vi "PurePursuit.vi"(0 "PathData":T2={"Path"=[{"x"=0.0, "y"=0.0}, {"x"=0.0, "y"=46.0}, {"x"=77.25, "y"=97.5}], "Spacing"=0.0, "DistancesToEnd"=[309.52253206522465, 306.5225388483889, 303.52254576348514, 300.5225494135135, 297.5225482930251, 294.5225431892043, 291.52253649479525, 288.5225309404311, 285.52252839669825, 282.52252922985826, 279.52253236801363, 276.5225359199274, 273.5225380077533, 270.5225374640896, 267.5225341651582, 264.5225289486152, 261.52252321975885, 258.52251843460203, 255.52251565052453, 252.52251527415513, 249.52251704698162, 246.52252022727612, 243.52252387624657, 240.5225271449837, 237.52252948071848, 234.5225307115883, 231.5225310121264, 228.5225307841412, 225.52253050297352, 222.52253057724883, 219.522531255923, 216.52253259658312, 213.5225344902357, 210.52253672481638, 207.52253906428678, 204.52254132188853, 201.52254341264756, 198.5225453787386, 195.52254738922483, 192.52254972128023, 189.5225527326013, 186.5225568345679, 183.5225624736694, 180.52257012582595, 177.52258030545136, 174.52259358906986, 171.52261065227918, 168.52263231879937, 165.52265962102405, 162.52269387257934, 159.52273675466557, 156.52279041923995, 153.52285761342083, 150.52294183093122, 147.52304749810799, 144.52318020416902, 141.5233469881785, 138.52355669860665, 135.52382044572104, 132.52415217017628, 129.52456938475245, 126.52509392552396, 123.52575388229783, 120.52658224756205, 117.52762599636499, 114.52893466674816, 111.5305811433295, 108.53265099247815, 105.5352499693053, 102.53851522329074, 99.54261858949184, 96.54777258499563, 93.55424339621041, 90.56236601643654, 87.57255952674781, 84.58534501572932, 81.60137180227034, 78.62143961905741, 75.64655567097594, 72.6779255489502, 69.71706974165639, 66.76578984976493, 63.82625595622302, 60.90103565379168, 57.99306437227732, 55.10557379235981, 52.24189700353533, 49.40502603383819, 46.59675379579783, 43.81612021857386, 41.056705992040605, 38.30212773163372, 35.53590323835957, 32.752089130751756, 29.950811925036337, 27.135602619179224, 24.311917874683846, 21.486403150766286, 18.666614193530503, 15.861028930660632, 13.07925664424869, 10.33239795871144, 7.633538890247935, 4.998382632368401, 2.4460384085185156, 0.0]}, 1 "SensorData":T3, 3 "Trackwidth":dbl=40.0 format="%#_13g", 5 "LookAhead":dbl=30.0, 9 "MaxVel":dbl=85.0, 11 "error in (no error)":errorcluster, 12 "Max Accel":dbl=65.0 format="%#_13g", 14 "Gains":T4={"FFV"=0.0088, "FFA"=0.0017, "Vel PID"={"P"=0.01, "I"=0.007, "D"=0.0}} {"Vel PID"."D" format="%.3f"; "Vel PID"."I" format="%.3f"; "Vel PID"."P" format="%.3f"}) -> (2 "Graph":cluster{cluster{"x":dbl, "y":dbl}[]}[](graph)=[{[{"x"=0.0, "y"=0.0}, {"x"=6.123233995736766e-17, "y"=1.0}, {"x"=1.2246467991473532e-16, "y"=2.0}, {"x"=1.8369701987210297e-16, "y"=3.0}, {"x"=2.4492935982947064e-16, "y"=4.0}, {"x"=3.061616997868383e-16, "y"=5.0}, {"x"=3.6739403974420594e-16, "y"=6.0}, {"x"=4.286263797015736e-16, "y"=7.0}, {"x"=4.898587196589413e-16, "y"=8.0}, {"x"=5.51091059616309e-16, "y"=9.0}, {"x"=6.123233995736766e-16, "y"=10.0}, {"x"=6.735557395310443e-16, "y"=11.0}, {"x"=7.347880794884119e-16, "y"=12.0}, {"x"=7.960204194457795e-16, "y"=13.0}, {"x"=8.572527594031472e-16, "y"=14.0}, {"x"=9.18485099360515e-16, "y"=15.0}, {"x"=9.797174393178826e-16, "y"=16.0}, {"x"=1.0409497792752501e-15, "y"=17.0}, {"x"=1.102182119232618e-15, "y"=18.0}, {"x"=1.1634144591899855e-15, "y"=19.0}, {"x"=1.2246467991473533e-15, "y"=20.0}, {"x"=1.2858791391047208e-15, "y"=21.0}, {"x"=1.3471114790620886e-15, "y"=22.0}, {"x"=1.4083438190194562e-15, "y"=23.0}, {"x"=1.4695761589768238e-15, "y"=24.0}, {"x"=1.5308084989341915e-15, "y"=25.0}, {"x"=1.592040838891559e-15, "y"=26.0}, {"x"=1.6532731788489269e-15, "y"=27.0}, {"x"=1.7145055188062944e-15, "y"=28.0}, {"x"=1.7757378587636622e-15, "y"=29.0}, {"x"=1.83697019872103e-15, "y"=30.0}, {"x"=1.8982025386783976e-15, "y"=31.0}, {"x"=1.959434878635765e-15, "y"=32.0}, {"x"=2.0206672185931327e-15, "y"=33.0}, {"x"=2.0818995585505003e-15, "y"=34.0}, {"x"=2.1431318985078682e-15, "y"=35.0}, {"x"=2.204364238465236e-15, "y"=36.0}, {"x"=2.2655965784226034e-15, "y"=37.0}, {"x"=2.326828918379971e-15, "y"=38.0}, {"x"=2.388061258337339e-15, "y"=39.0}, {"x"=2.4492935982947065e-15, "y"=40.0}, {"x"=2.510525938252074e-15, "y"=41.0}, {"x"=2.5717582782094417e-15, "y"=42.0}, {"x"=2.6329906181668092e-15, "y"=43.0}, {"x"=2.6942229581241772e-15, "y"=44.0}, {"x"=2.7554552980815448e-15, "y"=45.0}, {"x"=0.0, "y"=46.0}, {"x"=0.8320502943378437, "y"=46.55470019622523}, {"x"=1.6641005886756874, "y"=47.10940039245046}, {"x"=2.4961508830135313, "y"=47.66410058867569}, {"x"=3.328201177351375, "y"=48.218800784900914}, {"x"=4.160251471689219, "y"=48.77350098112615}, {"x"=4.9923017660270625, "y"=49.328201177351374}, {"x"=5.824352060364906, "y"=49.8829013735766}, {"x"=6.65640235470275, "y"=50.437601569801835}, {"x"=7.488452649040593, "y"=50.99230176602706}, {"x"=8.320502943378438, "y"=51.54700196225229}, {"x"=9.152553237716281, "y"=52.10170215847752}, {"x"=9.984603532054125, "y"=52.65640235470275}, {"x"=10.816653826391969, "y"=53.211102550927976}, {"x"=11.648704120729812, "y"=53.76580274715321}, {"x"=12.480754415067656, "y"=54.320502943378436}, {"x"=13.3128047094055, "y"=54.87520313960366}, {"x"=14.144855003743343, "y"=55.4299033358289}, {"x"=14.976905298081187, "y"=55.98460353205412}, {"x"=15.80895559241903, "y"=56.53930372827935}, {"x"=16.641005886756876, "y"=57.09400392450458}, {"x"=17.47305618109472, "y"=57.64870412072981}, {"x"=18.305106475432563, "y"=58.20340431695504}, {"x"=19.137156769770407, "y"=58.75810451318027}, {"x"=19.96920706410825, "y"=59.3128047094055}, {"x"=20.801257358446094, "y"=59.867504905630724}, {"x"=21.633307652783937, "y"=60.42220510185595}, {"x"=22.46535794712178, "y"=60.976905298081185}, {"x"=23.297408241459625, "y"=61.53160549430641}, {"x"=24.12945853579747, "y"=62.086305690531645}, {"x"=24.961508830135312, "y"=62.64100588675687}, {"x"=25.793559124473155, "y"=63.1957060829821}, {"x"=26.625609418811, "y"=63.750406279207326}, {"x"=27.457659713148843, "y"=64.30510647543255}, {"x"=28.289710007486686, "y"=64.8598066716578}, {"x"=29.12176030182453, "y"=65.41450686788302}, {"x"=29.953810596162374, "y"=65.96920706410825}, {"x"=30.785860890500217, "y"=66.52390726033347}, {"x"=31.61791118483806, "y"=67.0786074565587}, {"x"=32.449961479175904, "y"=67.63330765278394}, {"x"=33.28201177351375, "y"=68.18800784900915}, {"x"=34.11406206785159, "y"=68.7427080452344}, {"x"=34.94611236218944, "y"=69.29740824145962}, {"x"=35.77816265652728, "y"=69.85210843768485}, {"x"=36.610212950865126, "y"=70.40680863391007}, {"x"=37.442263245202966, "y"=70.9615088301353}, {"x"=38.27431353954081, "y"=71.51620902636054}, {"x"=39.10636383387865, "y"=72.07090922258577}, {"x"=39.9384141282165, "y"=72.625609418811}, {"x"=40.77046442255434, "y"=73.18030961503622}, {"x"=41.60251471689219, "y"=73.73500981126145}, {"x"=42.43456501123003, "y"=74.28971000748668}, {"x"=43.266615305567875, "y"=74.8444102037119}, {"x"=44.098665599905715, "y"=75.39911039993714}, {"x"=44.93071589424356, "y"=75.95381059616237}, {"x"=45.7627661885814, "y"=76.5085107923876}, {"x"=46.59481648291925, "y"=77.06321098861282}, {"x"=47.42686677725709, "y"=77.61791118483805}, {"x"=48.25891707159494, "y"=78.17261138106329}, {"x"=49.09096736593278, "y"=78.7273115772885}, {"x"=49.923017660270624, "y"=79.28201177351374}, {"x"=50.755067954608464, "y"=79.83671196973897}, {"x"=51.58711824894631, "y"=80.3914121659642}, {"x"=52.41916854328415, "y"=80.94611236218944}, {"x"=53.251218837622, "y"=81.50081255841465}, {"x"=54.083269131959845, "y"=82.05551275463989}, {"x"=54.915319426297685, "y"=82.61021295086512}, {"x"=55.74736972063553, "y"=83.16491314709035}, {"x"=56.57942001497337, "y"=83.71961334331557}, {"x"=57.41147030931122, "y"=84.2743135395408}, {"x"=58.24352060364906, "y"=84.82901373576604}, {"x"=59.07557089798691, "y"=85.38371393199125}, {"x"=59.90762119232475, "y"=85.9384141282165}, {"x"=60.739671486662594, "y"=86.49311432444172}, {"x"=61.571721781000434, "y"=87.04781452066695}, {"x"=62.40377207533828, "y"=87.60251471689219}, {"x"=63.23582236967612, "y"=88.1572149131174}, {"x"=64.06787266401396, "y"=88.71191510934264}, {"x"=64.89992295835181, "y"=89.26661530556787}, {"x"=65.73197325268966, "y"=89.8213155017931}, {"x"=66.5640235470275, "y"=90.37601569801832}, {"x"=67.39607384136534, "y"=90.93071589424355}, {"x"=68.22812413570318, "y"=91.48541609046879}, {"x"=69.06017443004103, "y"=92.040116286694}, {"x"=69.89222472437888, "y"=92.59481648291924}, {"x"=70.72427501871671, "y"=93.14951667914447}, {"x"=71.55632531305456, "y"=93.7042168753697}, {"x"=72.3883756073924, "y"=94.25891707159494}, {"x"=73.22042590173025, "y"=94.81361726782015}, {"x"=74.05247619606808, "y"=95.36831746404539}, {"x"=74.88452649040593, "y"=95.92301766027062}, {"x"=75.71657678474378, "y"=96.47771785649584}, {"x"=76.54862707908163, "y"=97.03241805272107}, {"x"=77.25, "y"=97.5}]}, {[{"x"=77.17737509961091, "y"=96.61921805961741}, {"x"=87.19208931316219, "y"=103.23023153872136}]}, {[{"x"=77.25, "y"=97.5}]}, {[{"x"=106.17737509961091, "y"=96.61921805961741}, {"x"=104.75801407217037, "y"=105.58071089649088}, {"x"=100.63886793648439, "y"=113.66499037609913}, {"x"=94.22314741609263, "y"=120.08071089649088}, {"x"=86.13886793648439, "y"=124.19985703217687}, {"x"=77.17737509961091, "y"=125.61921805961741}, {"x"=68.21588226273744, "y"=124.19985703217687}, {"x"=60.131602783129196, "y"=120.08071089649088}, {"x"=53.71588226273744, "y"=113.66499037609913}, {"x"=49.59673612705146, "y"=105.58071089649088}, {"x"=48.17737509961091, "y"=96.61921805961741}, {"x"=49.59673612705146, "y"=87.65772522274393}, {"x"=53.71588226273744, "y"=79.5734457431357}, {"x"=60.13160278312919, "y"=73.15772522274393}, {"x"=68.21588226273744, "y"=69.03857908705795}, {"x"=77.17737509961091, "y"=67.61921805961741}, {"x"=86.13886793648439, "y"=69.03857908705795}, {"x"=94.22314741609263, "y"=73.15772522274393}, {"x"=100.63886793648439, "y"=79.57344574313568}, {"x"=104.75801407217037, "y"=87.65772522274393}, {"x"=106.17737509961091, "y"=96.61921805961741}]}, {[{"x"=-861.1099608069076, "y"=601.5180796852112}, {"x"=-831.4997189012965, "y"=414.5663700037659}, {"x"=-745.5674499688715, "y"=245.9147962350945}, {"x"=-611.7248032180614, "y"=112.07214948428447}, {"x"=-443.07322944939017, "y"=26.13988055185939}, {"x"=-256.12151976794485, "y"=-3.470361353751514}, {"x"=-69.1698100864995, "y"=26.13988055185939}, {"x"=99.48176368217185, "y"=112.07214948428447}, {"x"=233.3244104329819, "y"=245.9147962350944}, {"x"=319.256679365407, "y"=414.56637000376577}, {"x"=348.86692127101793, "y"=601.5180796852111}, {"x"=319.256679365407, "y"=788.4697893666564}, {"x"=233.324410432982, "y"=957.1213631353278}, {"x"=99.48176368217202, "y"=1090.9640098861378}, {"x"=-69.16981008649935, "y"=1176.8962788185631}, {"x"=-256.1215197679447, "y"=1206.506520724174}, {"x"=-443.07322944939006, "y"=1176.8962788185631}, {"x"=-611.7248032180614, "y"=1090.964009886138}, {"x"=-745.5674499688714, "y"=957.121363135328}, {"x"=-831.4997189012965, "y"=788.4697893666566}, {"x"=-861.1099608069076, "y"=601.5180796852113}]}], 4 "LeftValue":dbl, 6 "RightValue":dbl, 10 "Done":bool, 15 "error out":errorcluster)   [LabVIEW 2017]
doc: "Takes in encoder and gyro data, and a path. In real time, calculates the left and right power to send to the motors to travel the path at a specified max speed, acceleration, and lookahead distance"
panel:
  out "Waveform Chart":T1(graph)
  in  "Average Vels":bool
  # "SET DEFAULTS"
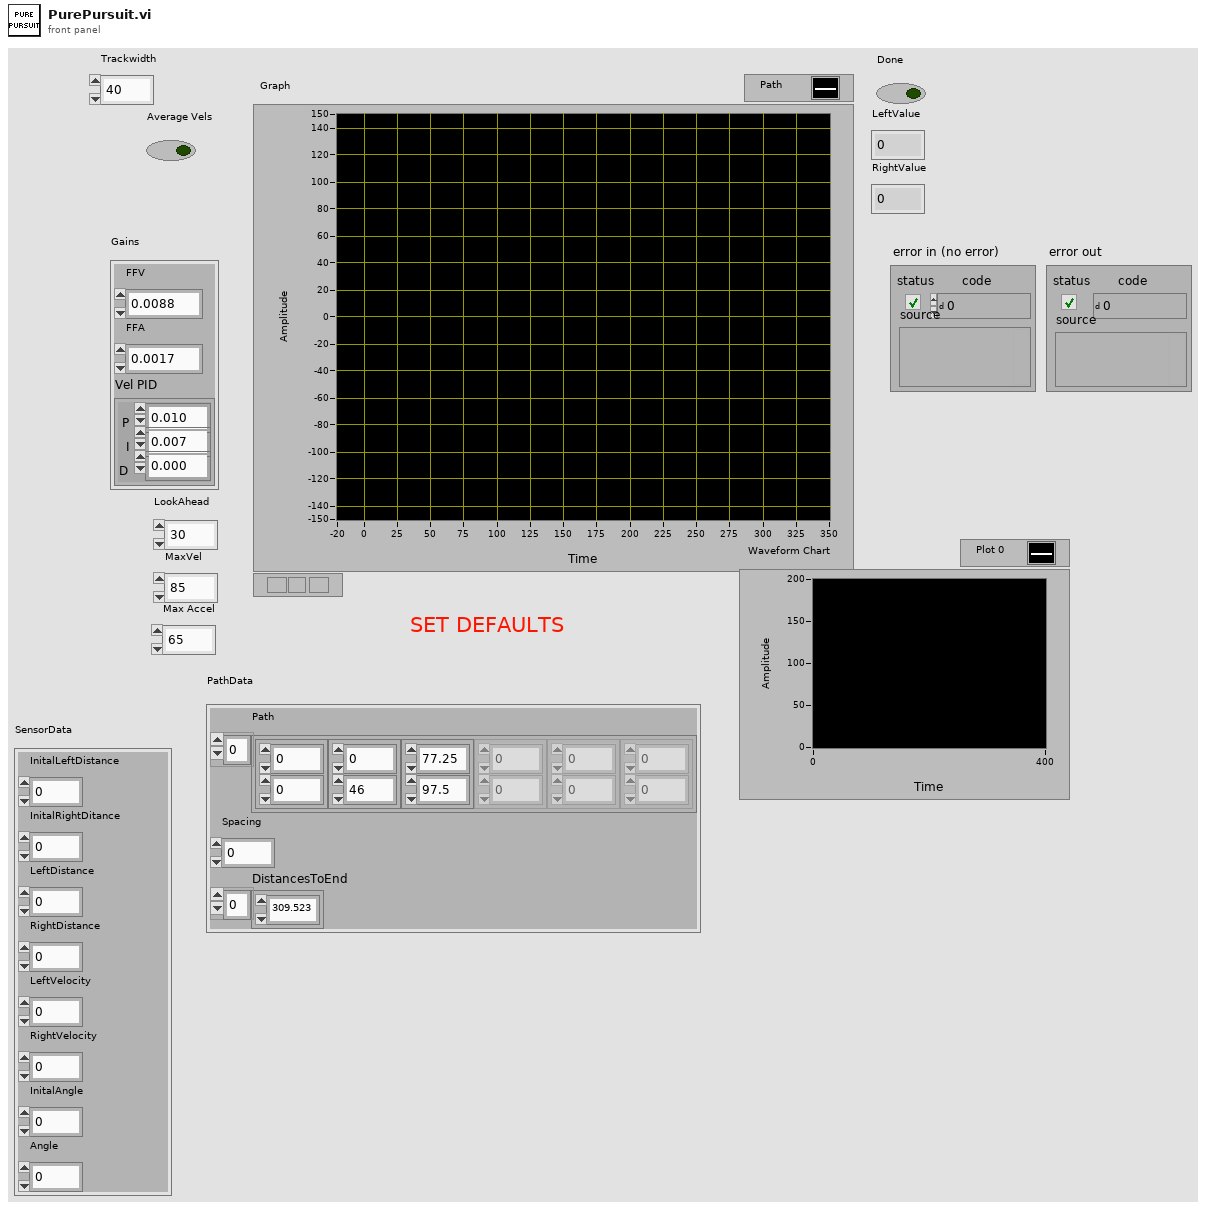
[diagram p1: front panel]
types:
  T1 = cluster{"l":dbl, "dx/dt":dbl, "r":dbl, "dx/dt":dbl}
  T2 = cluster{"Path":cluster{"x":dbl, "y":dbl}[], "Spacing":dbl, "DistancesToEnd":dbl[]}
  T3 = cluster{"InitalLeftDistance":dbl, "InitalRightDitance":dbl, "LeftDistance":dbl, "RightDistance":dbl, "LeftVelocity":dbl, "RightVelocity":dbl, "InitalAngle":dbl, "Angle":dbl}
  T4 = cluster{"FFV":dbl, "FFA":dbl, "Vel PID":cluster{"P":dbl, "I":dbl, "D":dbl}}
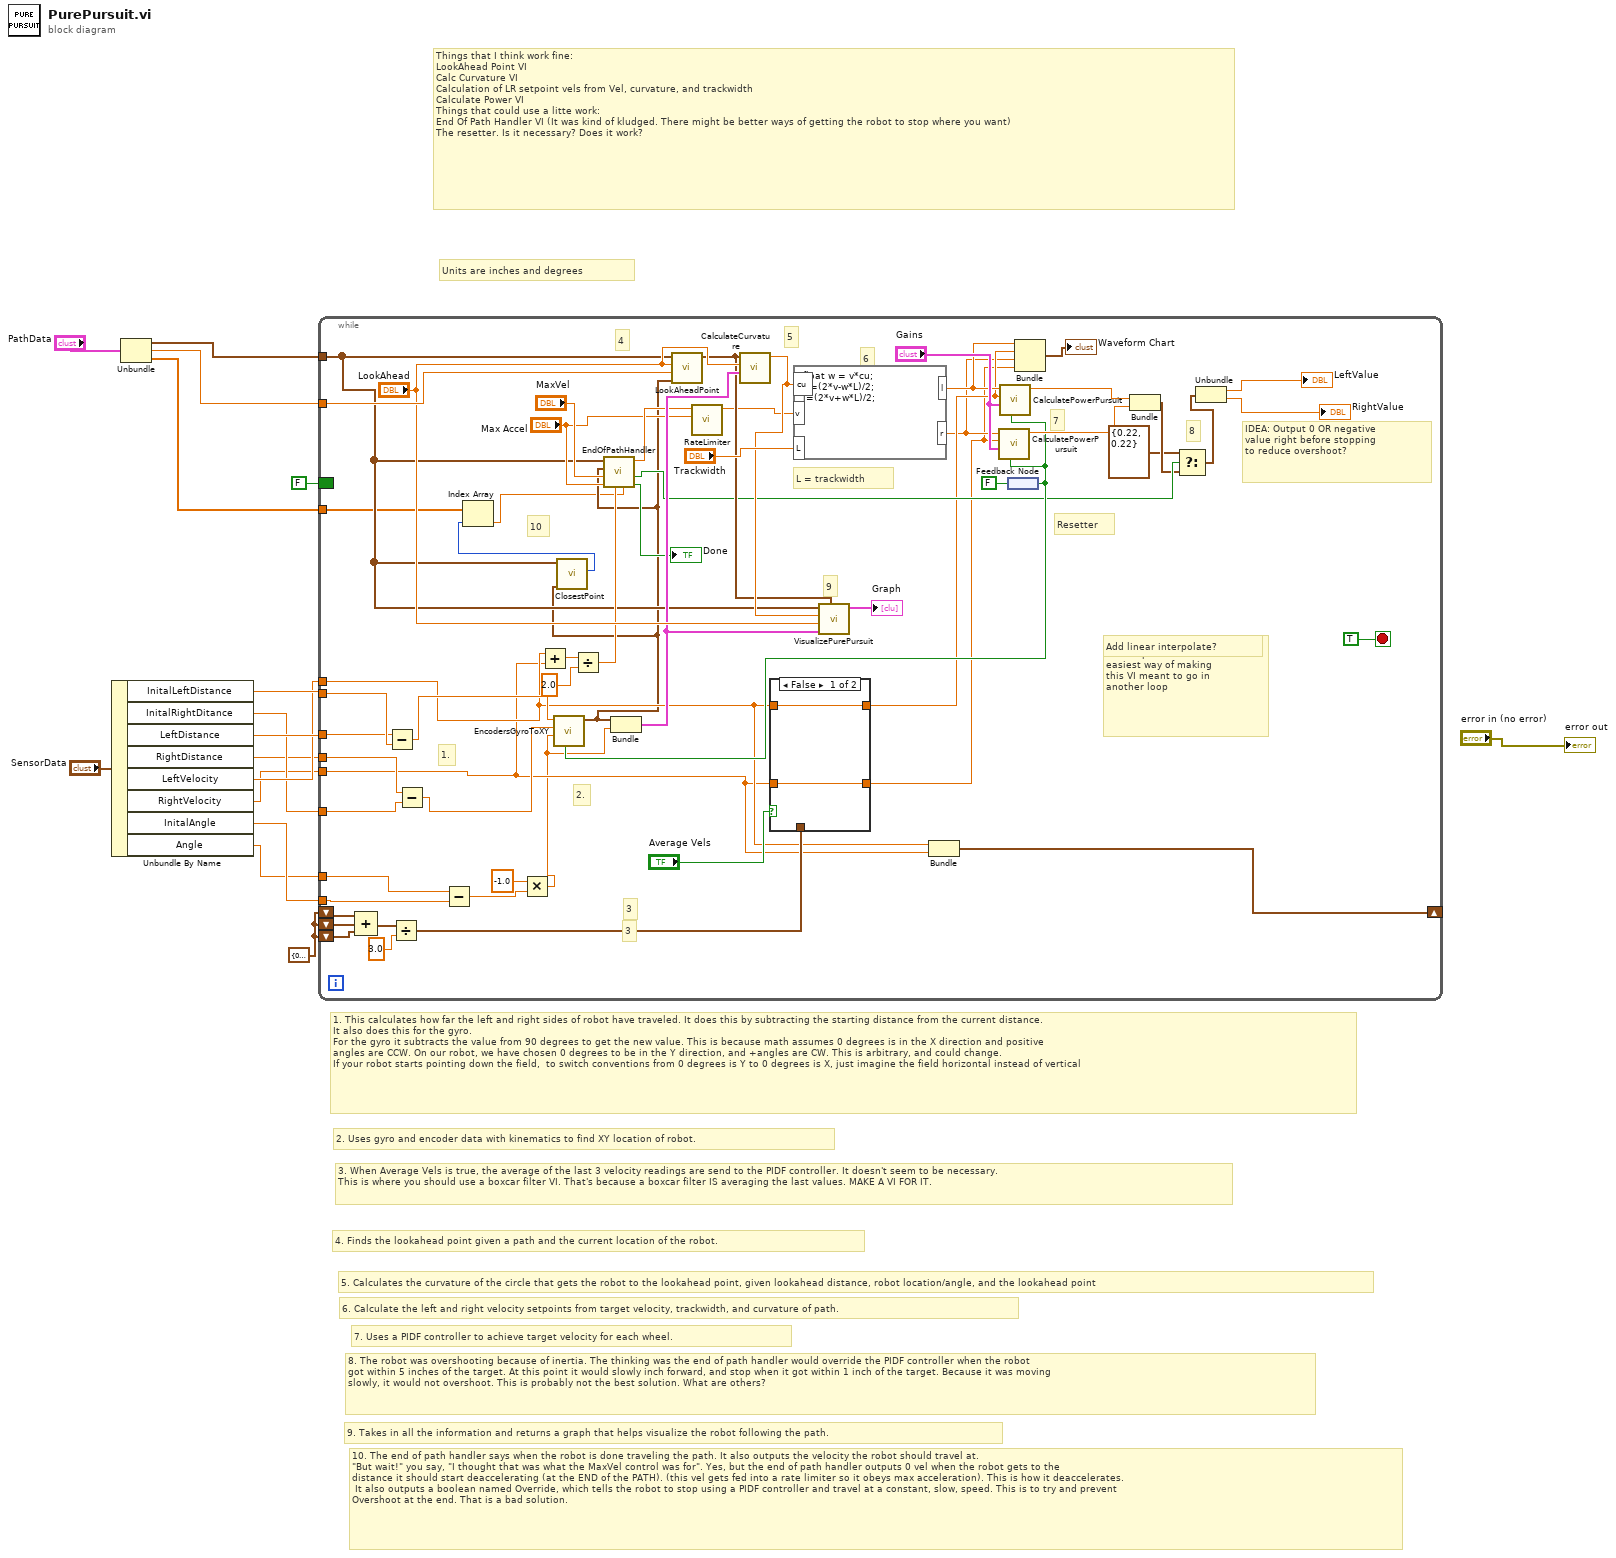
[diagram p0: block diagram]
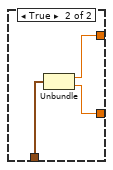
[diagram p2: hidden frame]
diagram:
  w16 = cluster{"dx/dt":dbl, "dx/dt":dbl} {"dx/dt"=0.0, "dx/dt"=0.0}
  # "10. The end of path handler says when the robot is done traveling the path. It also outputs the velocity the robot should travel at.\n\"But wait!\" you say, \"I thought that was what the MaxVel control was for\". Yes, but the end of path handler outputs 0 vel when the robot gets to the\ndistance it should start deaccelerating (at the END of the PATH). (this vel gets fed into a rate limiter so it obeys max acceleration). This is how it deaccelerates. \n It also outputs a boolean named Override, which tells the robot to stop using a PIDF controller and travel at a constant, slow, speed. This is to try and prevent\nOvershoot at the end. That is a bad solution."
  # "9. Takes in all the information and returns a graph that helps visualize the robot following the path."
  # "8. The robot was overshooting because of inertia. The thinking was the end of path handler would override the PIDF controller when the robot\ngot within 5 inches of the target. At this point it would slowly inch forward, and stop when it got within 1 inch of the target. Because it was moving\nslowly, it would not overshoot. This is probably not the best solution. What are others?"
  # "7. Uses a PIDF controller to achieve target velocity for each wheel."
  # "6. Calculate the left and right velocity setpoints from target velocity, trackwidth, and curvature of path."
  # "Things that I think work fine:\nLookAhead Point VI\nCalc Curvature VI\nCalculation of LR setpoint vels from Vel, curvature, and trackwidth\nCalculate Power VI\nThings that could use a litte work:\nEnd Of Path Handler VI (It was kind of kludged. There might be better ways of getting the robot to stop where you want)\nThe resetter. Is it necessary? Does it work?"
  # "Units are inches and degrees"
  # "5. Calculates the curvature of the circle that gets the robot to the lookahead point, given lookahead distance, robot location/angle, and the lookahead point"
  # "4. Finds the lookahead point given a path and the current location of the robot."
  # "3. When Average Vels is true, the average of the last 3 velocity readings are send to the PIDF controller. It doesn't seem to be necessary.\nThis is where you should use a boxcar filter VI. That's because a boxcar filter IS averaging the last values. MAKE A VI FOR IT."
  # "2. Uses gyro and encoder data with kinematics to find XY location of robot."
  # "1. This calculates how far the left and right sides of robot have traveled. It does this by subtracting the starting distance from the current distance.\nIt also does this for the gyro.\nFor the gyro it subtracts the value from 90 degrees to get the new value. This is because math assumes 0 degrees is in the X direction and positive\nangles are CCW. On our robot, we have chosen 0 degrees to be in the Y direction, and +angles are CW. This is arbitrary, and could change.\nIf your robot starts pointing down the field,  to switch conventions from 0 degrees is Y to 0 degrees is X, just imagine the field horizontal instead of vertical"
  n1 = Unbundle By Name("SensorData") -> ("InitalLeftDistance"=w12:dbl, "InitalRightDitance"=w9:dbl, "LeftDistance"=w11:dbl, "RightDistance"=w8:dbl, "LeftVelocity"=w10:dbl, "RightVelocity"=w7:dbl, "InitalAngle"=w6:dbl, "Angle"=w5:dbl)
  n2 = Unbundle("PathData") -> ("Path"=w3:cluster{"x":dbl, "y":dbl}[], "Spacing"=w2:dbl, "DistancesToEnd"=w1:dbl[])
  n3 = while {
    tunnel: w3 -> [w22]
    tunnel: w2 -> [w73]
    shift-right: [w65] -> _
    shift-left: w16 -> [w64]
    shift-left: w16 -> [w63]
    shift-left: w16 -> [w62]
    border: FALSE ("ENABLE") -> [_]
    tunnel: w6 -> [w51]
    tunnel: w9 -> [w50]
    tunnel: w12 -> [w49]
    tunnel: w11 -> [w35]
    tunnel: w10 -> [w34]
    tunnel: w8 -> [w33]
    tunnel: w7 -> [w32]
    tunnel: w5 -> [w31]
    tunnel: w1 -> [w19]
    stop <- TRUE stop-if-true
    # "IDEA: Output 0 OR negative\nvalue right before stopping\nto reduce overshoot?"
    # "10"
    # "9"
    # "8"
    # "7"
    # "6"
    # "5"
    # "4"
    # "3"
    # "3"
    # "2."
    # "1."
    # "I already had everything\nin a loop so this was the\neasiest way of making\nthis VI meant to go in\nanother loop"
    # "Resetter"
    # "Add linear interpolate?"
    # "L = trackwidth"
    n4 = Compound Arithmetic op=ADD(w64, w63, w62) -> (w61:cluster{"dx/dt":dbl, "dx/dt":dbl})
    n5 = Subtract(x=w35, y=w49) -> (x-y=w70:dbl)
    n6 = Divide(x=w61, y=3.0 ("x")) -> (x/y=w58:cluster{"dx/dt":dbl, "dx/dt":dbl})
    n7 = Subtract(x=w33, y=w50) -> (x-y=w74:dbl)
    n8 = Subtract(x=w31, y=w51) -> (x-y=w25:dbl)
    n9 = Multiply(x=-1.0, y=w25) -> (x*y=w27:dbl)
    n10 = Add(x=w34, y=w32) -> (x+y=w41:dbl)
    n11 = Divide(x=w41, y=2.0) -> (x/y=w39:dbl)
    n12 = case shown="False" "Average Vels" {
      tunnel: w32 -> [w76 _]
      tunnel: [w76 w78] -> w23
      tunnel: w34 -> [w75 _]
      tunnel: [w75 w79] -> w28
      tunnel: w58 -> [_ w77]
      frame False {
      }
      frame True {
        n13 = Unbundle(w77) -> ("dx/dt"=w79:dbl, "dx/dt"=w78:dbl)
      }
    }
    n14 = Bundle("LeftVelocity"=w34, "RightVelocity"=w32) -> (w65:cluster{"LeftVelocity":dbl, "RightVelocity":dbl})  [unwired: 1 in]
    n15 = feedback-in #1(FALSE ("ENABLE")) -> ()
    n16 = feedback #1() -> (w54:bool)
    n17 = call "EncodersGyroToXY.vi"("Reset"=w54, "Angle (degrees)"=w27, "Right Distance"=w74, "Left Distance"=w70) -> ("Location"=w21:cluster{dbl, dbl})  [unwired: 6 in, 1 out]
    n18 = call "ClosestPoint.vi"("Robot"=w21, "Path"=w22) -> ("ClosestIndex"=w18:i32)  [unwired: 8 in, 1 out]
    n19 = Index Array(array=w19, index=w18) -> (element=w17:dbl)
    n20 = call "EndOfPathHandler.vi"("DistanceToEnd"=w17, "CurrentVel"=w39, "MaxAccel"="Max Accel", "MaxVel"="MaxVel", "RobotLocation"=w21, "Path"=w22) -> ("Done"=→"Done":bool, "Override"=w45:bool, "VelOut"=w48:dbl)  [unwired: 2 in, 1 out]
    n21 = Bundle("Location"=w21, w27) -> (w67:cluster{"Location":cluster{dbl, dbl}, dbl})  [unwired: 1 in]
    n22 = call "LookAheadPoint.vi"("Robot"=w21, "Spacing"=w73, "LookAhead"="LookAhead", "Path"=w22) -> ("Point"=w66:cluster{"x":dbl, "y":dbl})  [unwired: 6 in, 1 out]
    n23 = call "RateLimiter.vi"("Max dx/dt"="Max Accel", "Input"=w48) -> ("Output"=w46:dbl)  [unwired: 9 in]
    n24 = call "CalculateCurvature.vi"("Robot"=w67, "Lookahead"="LookAhead", "Point"=w66) -> ("Curvature"=w69:dbl)  [unwired: 8 in]
    n25 = formula code="float w = v*cu;\nr =(2*v-w*L)/2;\nl=(2*v+w*L)/2;"("L"="Trackwidth", "cu"=w69, "v"=w46) -> ("r"=w24:dbl, "l"=w30:dbl)
    n26 = call "VisualizePurePursuit.vi"("Lookahead Point"=w66, "Robot"=w67, "Lookahead"="LookAhead", "Curvature"=w69, "Path"=w22) -> ("Graph"=→"Graph":cluster{cluster{"x":dbl, "y":dbl}[]}[])  [unwired: 6 in]
    n27 = call "CalculatePowerPursuit.vi"("Reset"=w54, "Gains"="Gains", "Vel"=w23, "Target Vel"=w24) -> ("Power"=w56:dbl)  [unwired: 7 in]
    n28 = call "CalculatePowerPursuit.vi"("Reset"=w54, "Gains"="Gains", "Vel"=w28, "Target Vel"=w30) -> ("Power"=w57:dbl)  [unwired: 7 in]
    n29 = Bundle("l"=w30, "dx/dt"=w28, "r"=w24, "dx/dt"=w23) -> (→"Waveform Chart":T1)  [unwired: 1 in]
    n30 = Bundle("Power"=w57, "Power"=w56) -> (w44:cluster{"Power":dbl, "Power":dbl})  [unwired: 1 in]
    n31 = Select(t=cluster{"Power":dbl, "Power":dbl} {"Power"=0.22, "Power"=0.22}, s=w45, f=w44) -> (s? t:f=w42:cluster{"Power":dbl, "Power":dbl})
    n32 = Unbundle(w42) -> ("Power"=→"LeftValue":dbl, "Power"=→"RightValue":dbl)
  }
  "error out" <- "error in (no error)"
